vi "test.vi"() -> ()   [LabVIEW 2016]
uses:
  <vilib>/Instr/_visa.llb/VISA Open Access Mode.ctl
panel:
  in  "write buffer":string="ID?\n"
  out "read buffer":string
  out "error out":errorcluster
  in  "error in (no error)":errorcluster
  in  "VISA resource name":refnum<visa-resource-name>="COM9"
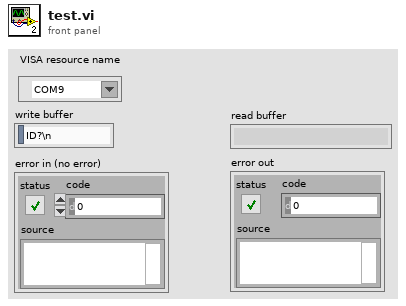
[diagram p1: front panel]
types:
  T1 = typedef "VISA Open Access Mode.ctl" = u32
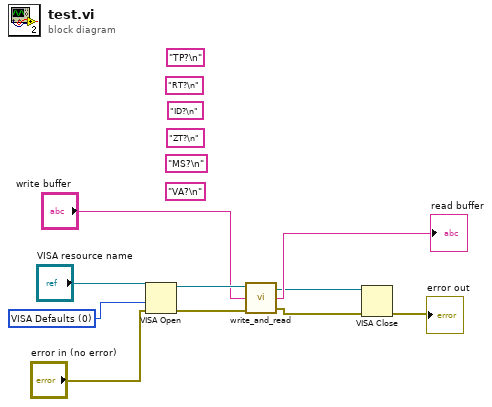
[diagram p0: block diagram]
diagram:
  (unwired) "VA?\n"
  (unwired) "TP?\n"
  (unwired) "RT?\n"
  (unwired) "MS?\n"
  (unwired) "ID?\n"
  (unwired) "ZT?\n"
  w8 = T1 0 items=["VISA Defaults"=0, "Exclusive Lock"=1, "Load Configured Settings"=4] ("Access Mode")
  n1 = VISA Open(access mode=w8, error in (no error)="error in (no error)", VISA resource name="VISA resource name") -> (VISA resource name=w7:refnum<visa-resource-name>, error out=w6:errorcluster)  [unwired: 2 in]
  n2 = call "write_and_read.vi"("error in"=w6, "write buffer"="write buffer", "VISA resource name in"=w7) -> ("error out"=w1:errorcluster, "read buffer"=→"read buffer":string, "VISA resource name out"=w2:refnum<visa-resource-name>)
  n3 = VISA Close(VISA resource name=w2, error in (no error)=w1) -> (error out=→"error out":errorcluster)
